vi "DWF MSO Init AtoD.vi"() -> (0 "Error Out":errorcluster, 3 "Instrument Handle Out":i32)   [LabVIEW 2025]
uses:
  <vilib>/DigilentWF/MSO/WF-MSO.lvlib
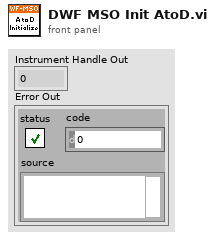
[diagram p1: front panel]
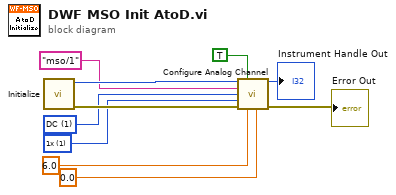
[diagram p0: block diagram]
diagram:
  w7 = 1 items=["AC", "DC"] ("Vertical Coupling")
  w8 = 1 items=["1x"=1, "10x"=10] ("Probe Attenuation")
  n1 = call <vilib>:"Initialize.vi"() -> ("Error Out"=w9:errorcluster, "Instrument Handle Out"=w10:i32)  [unwired: 10 in]
  n2 = call <vilib>:"Configure Analog Channel.vi"("Instrument Handle In"=w10, "Enable Channel"=TRUE, "Channel"="mso/1", "Vertical Coupling"=w7, "Probe Attenuation"=w8, "Error In"=w9, "Vertical Range"=6.0, "Vertical Offset"=0.0) -> ("Instrument Handle Out"=→"Instrument Handle Out":i32, "Error Out"=→"Error Out":errorcluster)  [unwired: 6 in]
